vi "E727_Absolute Move.vi"(0 "Target AbsolutePosition (um)":dbl[](array[numeric])=[150.0, 150.0] format="%.6f", 2 "StageChannels 2":string[](array[string]), 4 "stop 2":bool) -> (7 "Current position":dbl[](array[numeric]) format="%.6f", 9 "Pre-move position 2":dbl[](array[numeric]) format="%.6f")   [LabVIEW 2022 SP3]
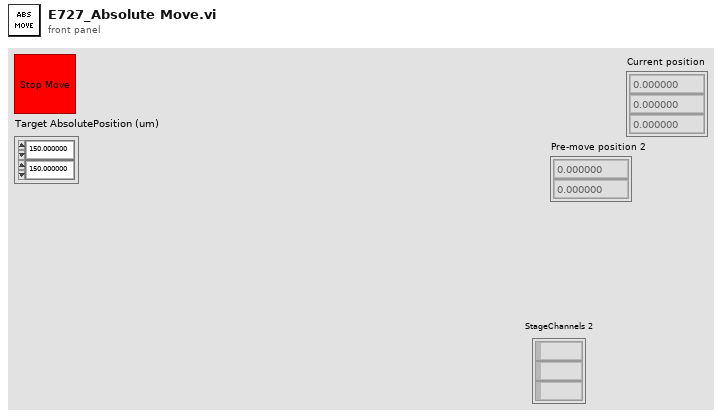
[diagram p1: front panel]
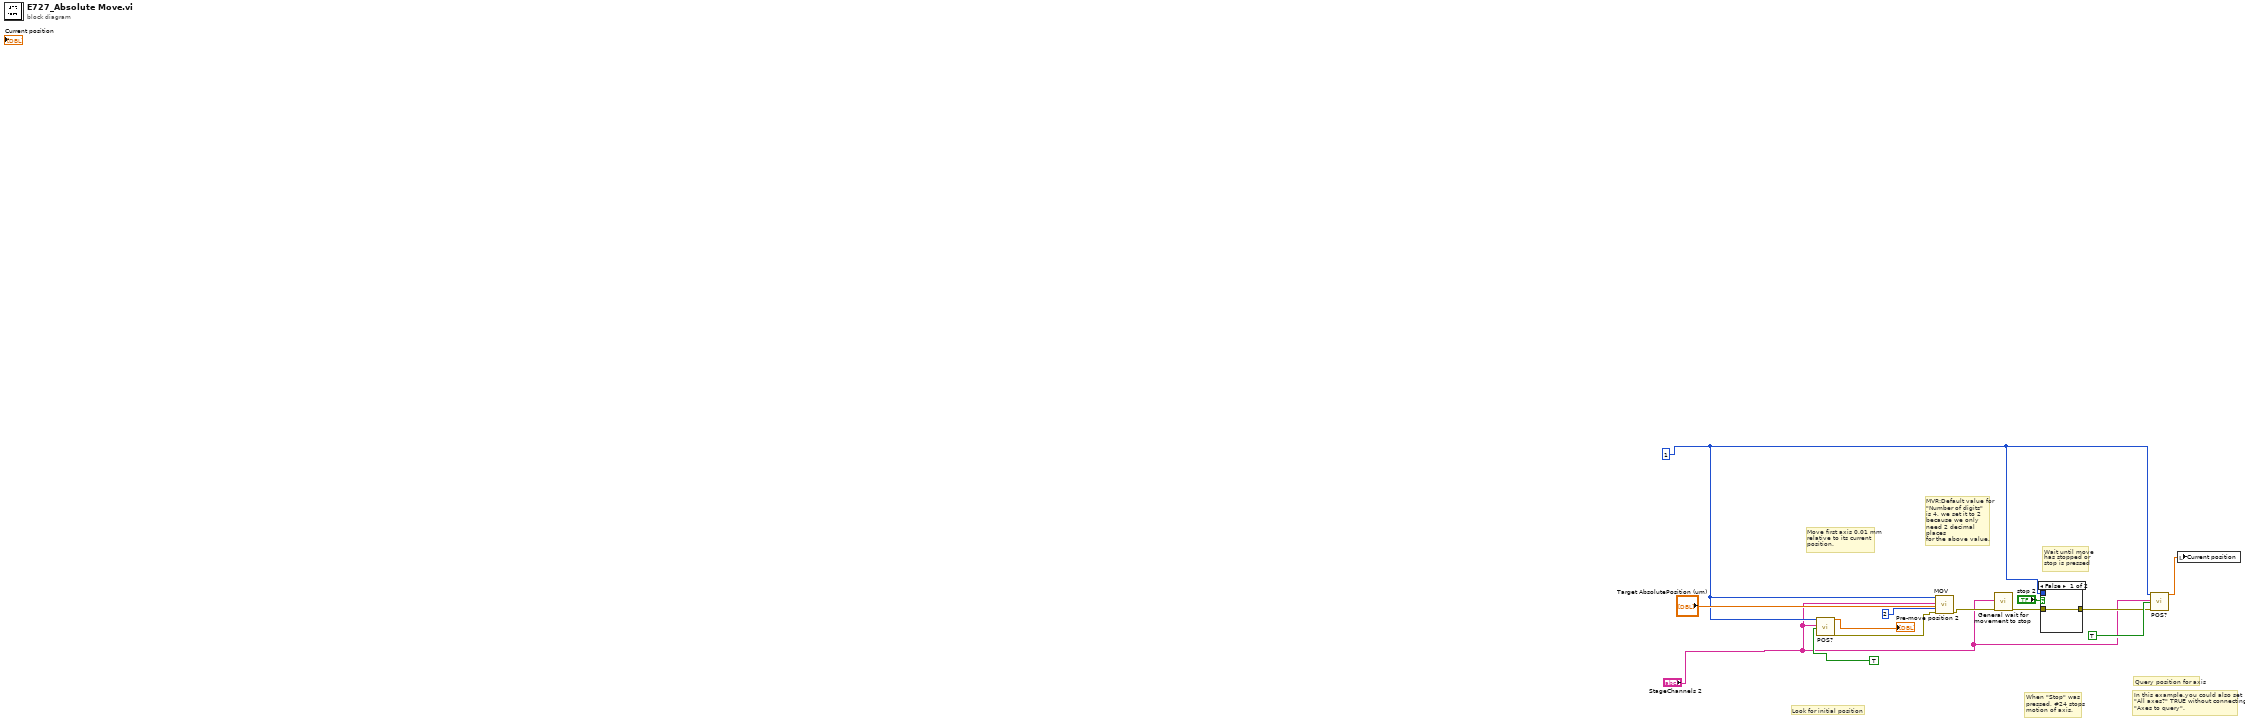
[diagram p0: block diagram]
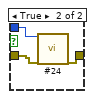
[diagram p2: hidden frame]
diagram:
  w2 = 1 ("System no.")
  # "Look for initial position"
  # "When \"Stop\" was \npressed, #24 stops\nmotion of axis."
  # "Wait until move\nhas stopped or\nstop is pressed"
  # "MVR:Default value for\n\"Number of digits\"\nis 4, we set it to 2\nbecause we only\nneed 2 decimal places\nfor the above value."
  # "Move first axis 0.01 mm\nrelative to its current\nposition."
  # "In this example,you could also set \n\"All axes?\" TRUE without connecting\n\"Axes to query\"."
  # "Query position for axis"
  n1 = call "POS?.vi"("System no."=w2, "Axes to query"="StageChannels 2", "All axes?"=TRUE) -> ("Position"=→"Pre-move position 2":dbl[], "error out"=w7:errorcluster)  [unwired: 2 in, 13 out]
  n2 = call "MOV.vi"("System no."=w2, "Axes to move"="StageChannels 2", "Position values"="Target AbsolutePosition (um)", "No.of digits"=i16 2, "error in"=w7) -> ("error out"=w6:errorcluster)  [unwired: 14 out]
  n3 = call "General wait for movement to stop.vi"("Axes to wait for"="StageChannels 2", "error in"=w6) -> ("error out"=w12:errorcluster)  [unwired: 6 in, 11 out]
  n4 = case shown="False" "stop 2" {
    tunnel: w12 -> [w14 w17]
    tunnel: [w14 w16] -> w11
    tunnel: w2 -> [_ w15]
    frame False {
    }
    frame True {
      n5 = call "#24.vi"("System no."=w15, "error in"=w17) -> ("error out"=w16:errorcluster)  [unwired: 17 out]
    }
  }
  n6 = call "POS?.vi"("System no."=w2, "Axes to query"="StageChannels 2", "All axes?"=TRUE, "error in"=w11) -> ("Position"=w3:dbl[])  [unwired: 1 in, 14 out]
  n7 = local write "Current position"(w3) -> ()
